vi "Queue Valid.vi"(8 "error in (no error)":errorcluster, 11 "queue name in":string) -> (0 "error out":errorcluster, 3 "invalid？":bool)   [LabVIEW 2023]
uses:
  Control/Queue Data.ctl
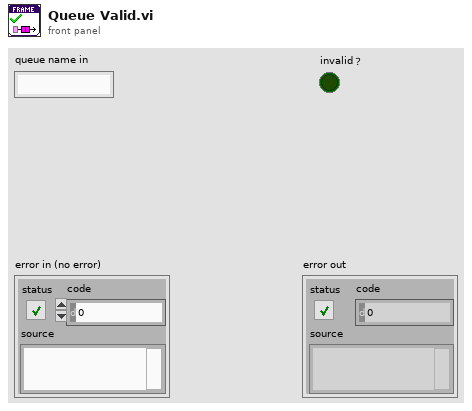
[diagram p1: front panel]
types:
  T1 = typedef "Queue Data.ctl" = cluster{"event":string, "data":variant}
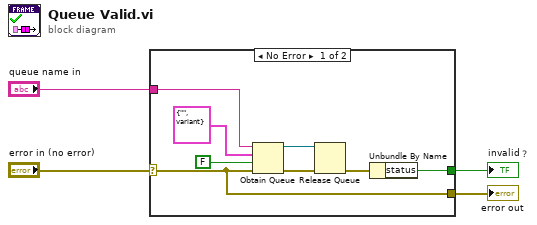
[diagram p0: block diagram]
diagram:
  n1 = case shown="No Error" "error in (no error)" {
    selector: "error in (no error)" -> [w9 w13]
    tunnel: [w9 w13] -> w3
    tunnel: "queue name in" -> [w10 _]
    tunnel: [w5 _] -> w1
    frame No Error {
      n2 = Obtain Queue(name (unnamed)=w10, element data type=T1 {"event"="", "data"=variant}, create if not found? (T)=FALSE, error in (no error)=w9) -> (queue out=w7:refnum<queue>, error out=w8:errorcluster)  [unwired: 1 in, 1 out]
      n3 = Release Queue(queue=w7, error in (no error)=w8) -> (error out=w6:errorcluster)  [unwired: 1 in, 2 out]
      n4 = Unbundle By Name(w6) -> ("status"=w5:bool)
    }
    frame Error {
    }
  }
  "error out" <- w3
  "invalid？" <- w1
